vi "GetSystemTime.vi"() -> ()   [LabVIEW 2018]
uses:
  Windows/System32/kernel32.dll
panel:
  in  "milliseconds to wait":u32
  in  "stop":bool
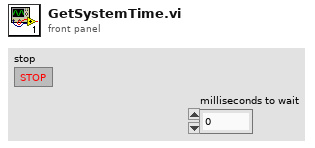
[diagram p1: front panel]
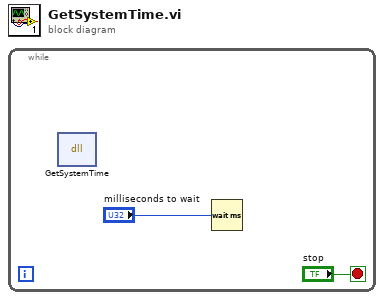
[diagram p0: block diagram]
diagram:
  n1 = while {
    stop <- "stop" stop-if-true
    n2 = dll-call lib="C:/Windows/System32/kernel32.dll" fn="GetSystemTime"() -> ()  [unwired: 6 in, 2 out]
    n3 = Wait (ms)(milliseconds to wait="milliseconds to wait") -> ()  [unwired: 1 out]
  }
